vi "LVFunction_Imop_Compute_ZernikePupil.vi"(0 "Pupil.lvclass":refnum<class "Pupil.lvclass">, 5 "center in":T1, 7 "radius in":sgl, 9 "CircularPupilDetectionParams":T2, 11 "error in":errorcluster) -> (4 "Pupil.lvclass":refnum<class "Pupil.lvclass">, 6 "center":T1, 8 "radius":sgl, 15 "error out":errorcluster)   [LabVIEW 2020]
doc: "Compute the geometric parameters of the Zernike pupil from a pupil input.\n\n<B>PupilIn</B> : pupil object.\n<B>PupilOut</B> : pupil object.\n<B>detection_mode</B> : E_PUPIL_DETECTION_T circular pupil detection mode.\n<B>covering</B> : E_PUPIL_COVERING_T circular pupil covering mode.\n<B>has_central_occultation</B> : If pupil has a central occultation, this boolean must be set to true to tell the circular pupil detector that internal sub-pupils are missing.\n<B>center</B> : User pupil center coordinates if detection mode = E_PUPIL_FIXED_CENTER. Value is ignore for other detection modes. Values are expressed in number of subpupils.\n<B>radius</B> : User pupil radius if detection mode = E_PUPIL_FIXED_RADIUS. Value is ignore for other detection modes. Value is expressed in number of subpupils.\n\n\n\nCompute the geometric parameters of the Zernike pupil from a cPupil input.\ndetection_mode\n Circular pupil detection mode enum. Detection mode must be set as follow: -\n detectionMode = 0 to fix radius and let detector find best center.\n * detectionMode = 1 to fix center and let detector find best radius.\n * detectionMode = 2 to let detector find best combination of radius and center.\n\ncovering\n circular pupil covering enum. Covering must be set as follows: - covering = 0\n inscribed to have detected pupil inscribed in measured pupil\n * covering = 1 circumscribed to have detected pupil circumscribed to measured\n\nhas_central_occultation\n If pupil has a central occultation, this boolean must be set to true to tell\n the circular pupil detector that internal sub-pupils are missing.\n\ncenter\n Pupil center pair in manual_center detection mode = 1. If detection_mode is\n not manual center, value is not taken into account.\n\nradius\n Pupil radius in manual radius detection mode detection mode = 0. If\n detection_mode is not manual radius, value is not taken into account."
uses:
  Pupil.lvclass
  CircularPupilDetectionParams.ctl
  PupilDetectionOption.ctl
  CircularAutoDetectionOptions.ctl
  PupilDetectionMode.ctl
  Point2Df.ctl
  LVClass_Pupil Read Pupil.vi
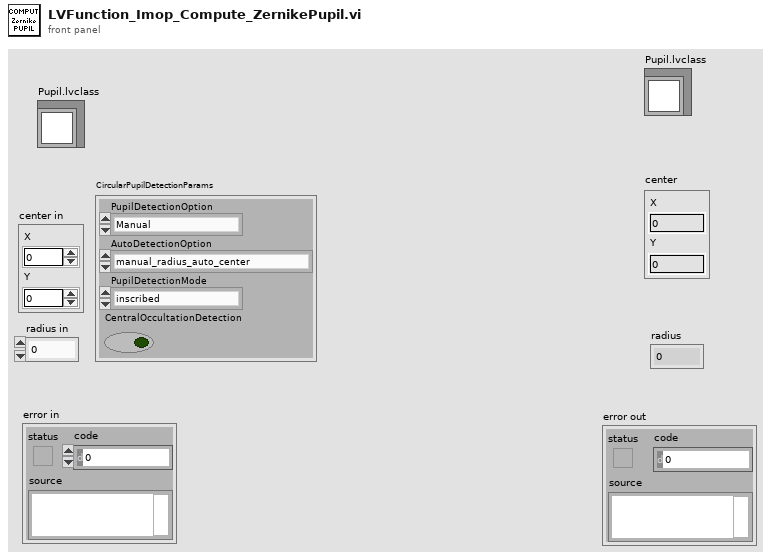
[diagram p1: front panel]
types:
  T1 = typedef "Point2Df.ctl" = cluster{"X":sgl, "Y":sgl}
  T2 = typedef "CircularPupilDetectionParams.ctl" = cluster{"PupilDetectionOption":T3, "AutoDetectionOption":T4, "PupilDetectionMode":T5, "CentralOccultationDetection":bool}
  T3 = typedef "PupilDetectionOption.ctl" = enum16{"Manual", "Automatic"}
  T4 = typedef "CircularAutoDetectionOptions.ctl" = enum16{"manual_radius_auto_center", "manual_center_auto_radius", "auto_radius_auto_center"}
  T5 = typedef "PupilDetectionMode.ctl" = enum16{"inscribed", "circumscribed"}
  T6 = typedef "ClassID.ctl" = i64
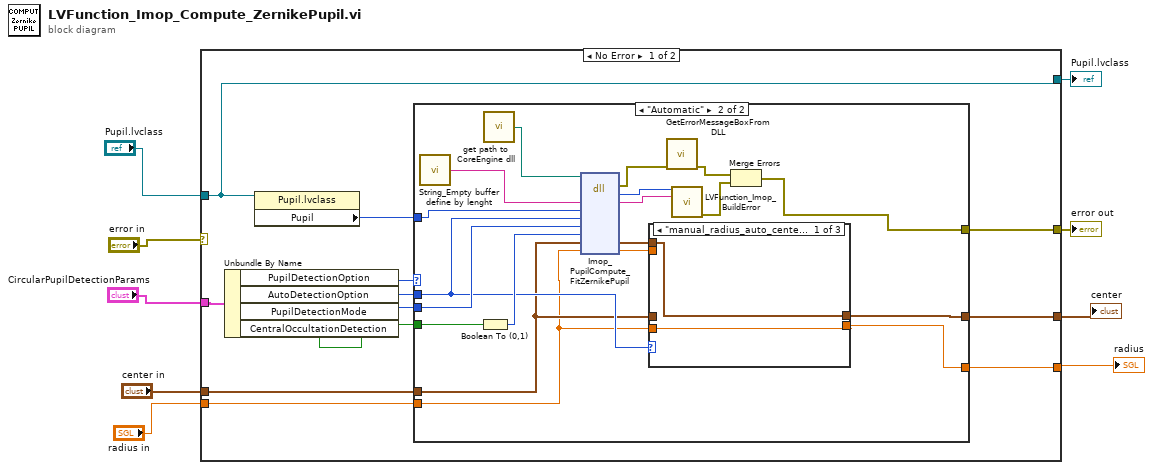
[diagram p0: block diagram]
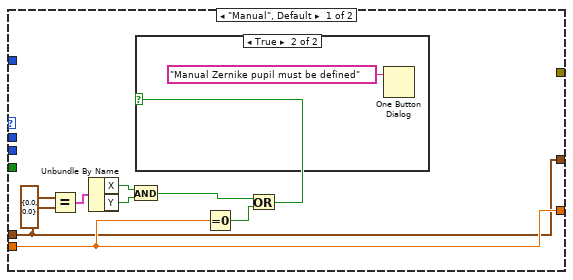
[diagram p2: hidden frame]
diagram:
  n1 = case shown="No Error" "error in" {
    selector: "error in" -> [_ w58]
    tunnel: "Pupil.lvclass" -> [w16 w57]
    tunnel: "CircularPupilDetectionParams" -> [w20 _]
    tunnel: [w17 w58] -> w6
    tunnel: [w16 w57] -> w5
    tunnel: [w15 _] -> w3
    tunnel: [w14 _] -> w4
    tunnel: "center in" -> [w12 _]
    tunnel: "radius in" -> [w11 _]
    frame No Error {
      n2 = Unbundle By Name(w20) -> ("PupilDetectionOption"=w13:T3, "AutoDetectionOption"=w10:T4, "PupilDetectionMode"=w19:T5, "CentralOccultationDetection"=w18:bool)
      n3 = property class="Pupil.lvclass"(reference=w16) -> ("Pupil"=w21:T6)  [unwired: 1 in, 2 out]
      n4 = case shown="\"Automatic\"" w13 {
        tunnel: w21 -> [_ w45]
        tunnel: w19 -> [_ w44]
        tunnel: w18 -> [_ w43]
        tunnel: [_ w32] -> w17
        tunnel: [w29 w39] -> w15
        tunnel: [w30 w37] -> w14
        tunnel: w12 -> [w29 w36]
        tunnel: w11 -> [w30 w35]
        tunnel: w10 -> [_ w41]
        frame "Manual", Default {
          n5 = Equal?(x=w29, y=T1 {"X"=0.0, "Y"=0.0}) -> (x = y?=w27:cluster{"X":bool, "Y":bool})
          n6 = Unbundle By Name(w27) -> ("X"=w26:bool, "Y"=w25:bool)
          n7 = And(x=w26, y=w25) -> (x .and. y?=w24:bool)
          n8 = Equal To 0?(x=w30) -> (x = 0?=w23:bool)
          n9 = Or(x=w24, y=w23) -> (x .or. y?=w22:bool)
          n10 = case shown="True" w22 {
            frame False {
            }
            frame True {
              n11 = One Button Dialog(message="Manual Zernike pupil must be defined") -> ()  [unwired: 1 in, 1 out]
            }
          }
        }
        frame "Automatic" {
          n12 = call "String_Empty buffer define by lenght.vi"() -> ("Empty buffer"=w50:string)  [unwired: 1 in]
          n13 = Boolean To (0,1)(Boolean=w43) -> (0, 1=w42:i16)
          n14 = call "get path to CoreEngine dll.vi"() -> ("path to wavekit library"=w47:path)  [unwired: 14 in, 1 out]
          n15 = dll-call lib="D:/FLE/0.Code/CoreEngine4_Suite/LV2011_interface/DLLs/c_interface_vc100.dll" fn="Imop_PupilCompute_FitZernikePupil"(path in=w47, "message"=w50, "Pupil"=w45, "AutoDetectionOption"=w41, "PupilDetectionMode"=w44, "CentralOccultationDetection"=w42, "center"=w36, "rayon"=w35) -> (error out=w46:errorcluster, "return type"=w48:i32, "message"=w49:string, "center"=w40:T1, "rayon"=w38:sgl)  [unwired: 6 in, 1 out]
          n16 = case shown="\"manual_radius_auto_center\", Default" w41 {
            tunnel: [w51 w53 w56] -> w39
            tunnel: w40 -> [w51 _ w56]
            tunnel: [w52 w54 w55] -> w37
            tunnel: w38 -> [_ w54 w55]
            tunnel: w36 -> [_ w53 _]
            tunnel: w35 -> [w52 _ _]
            frame "manual_radius_auto_center", Default {
            }
            frame "manual_center_auto_radius" {
            }
            frame "auto_radius_auto_center" {
            }
          }
          n17 = call "GetErrorMessageBoxFromDLL.vi"("error IN"=w46) -> ("error OUT"=w34:errorcluster)  [unwired: 10 in]
          n18 = call "LVFunction_Imop_BuildError.vi"("code"=w48, "String to Prepend to source (\"\")"=w49) -> ("error out"=w33:errorcluster)  [unwired: 13 in]
          n19 = Merge Errors(w34, w33) -> (w32:errorcluster)
        }
      }
    }
    frame Error {
    }
  }
  "error out" <- w6
  "Pupil.lvclass" <- w5
  "radius" <- w4
  "center" <- w3
